vi "Config Field.vi"(0 "VISA resource name":refnum<visa-resource-name>, 1 "Frequency  (7)":i32=7 min=0 max=7, 2 "Capacitance (9)":i32=9 min=0 max=9, 3 "Loss (9)":i32=9 min=0 max=9, 4 "Voltage (on)":enum16{"off", "on"}(ring)=enum."on", 5 "Atten (on)":enum16{"off", "on"}(ring)=enum."on", 6 "Error Messages (English)":i32(ring)=1 items=["Numeric", "English"], 7 "error in":errorcluster, 8 "Sample (off)":enum16{"off", "on"}(ring), 9 "Voltage Reduced  (2)":i32=2 min=0 max=2) -> (20 "VISA resource name out":refnum<visa-resource-name>, 27 "error out":errorcluster)   [LabVIEW 2019, in "Andeen-Hagerling 2700(400 firmware).lvlib"]
doc: "The FIELD command allows you to configure the seven fields in the result line that are sent to the remote system."
uses:
  Andeen-Hagerling 2700(400 firmware).lvlib
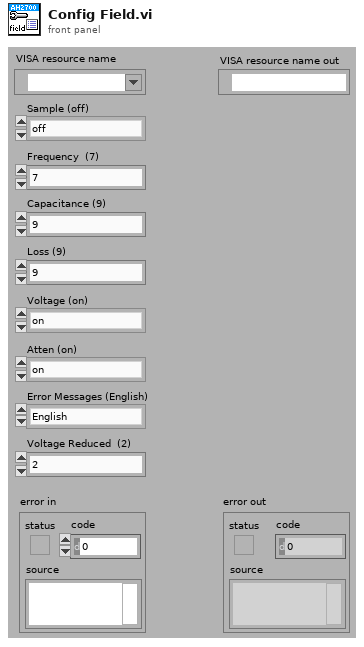
[diagram p1: front panel]
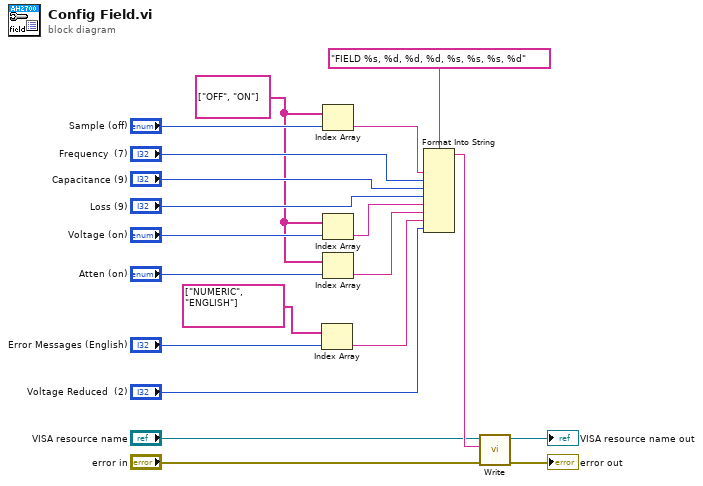
[diagram p0: block diagram]
diagram:
  w5 = string[] ["OFF", "ON"]
  n1 = Index Array(array=string[] ["NUMERIC", "ENGLISH"], index="Error Messages (English)") -> (element=w1:string)
  n2 = Index Array(array=w5, index="Sample (off)") -> (element=w9:string)
  n3 = Index Array(array=w5, index="Voltage (on)") -> (element=w8:string)
  n4 = Index Array(array=w5, index="Atten (on)") -> (element=w4:string)
  n5 = Format Into String(format string="FIELD %s, %d, %d, %d, %s, %s, %s, %d", w9, "Frequency  (7)", "Capacitance (9)", "Loss (9)", w8, w4, w1, "Voltage Reduced  (2)") -> (resulting string=w17:string)  [unwired: 2 in, 1 out]
  n6 = call "Write.vi"("error in"="error in", "command"=w17, "VISA resource name"="VISA resource name") -> ("error out"=→"error out":errorcluster, "VISA resource name out"=→"VISA resource name out":refnum<visa-resource-name>)  [unwired: 7 in]
